vi "Sort DPID IDs by Speed.vi"(11 "DPIDs":T2[](array[typedef])) -> (3 "Filtered DPIDs IDs":T1)   [LabVIEW 2013]
uses:
  DPID Parameters.ctl
  DPID Periodic Rate.ctl
  Filtered DPID IDs.ctl
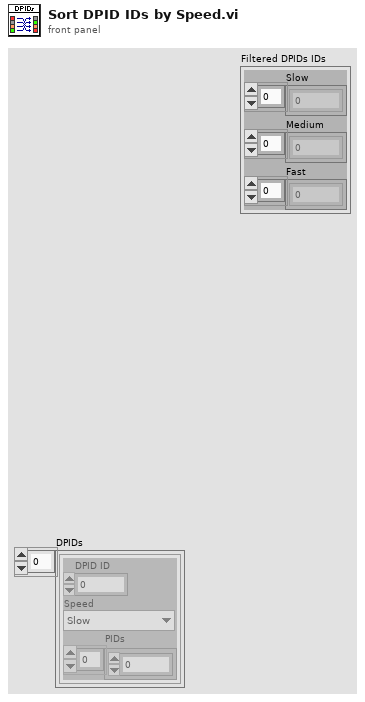
[diagram p1: front panel]
types:
  T1 = typedef "Filtered DPID IDs.ctl" = cluster{"Slow":u8[], "Medium":u8[], "Fast":u8[]}
  T2 = typedef "DPID Parameters.ctl" = cluster{"DPID ID":u8, "Speed":T3, "PIDs":u16[]}
  T3 = typedef "DPID Periodic Rate.ctl" = enum16{"Slow", "Medium", "Fast"}
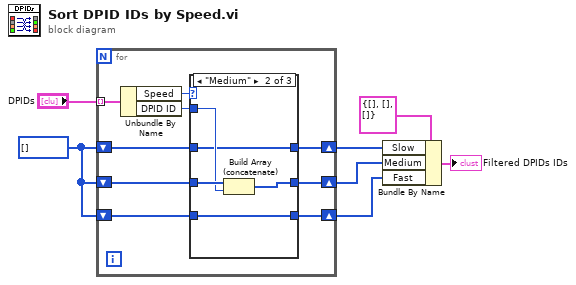
[diagram p0: block diagram]
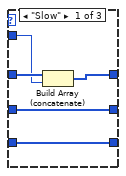
[diagram p2: hidden frame]
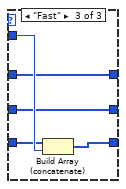
[diagram p3: hidden frame]
diagram:
  w6 = u8[] []
  n1 = for {
    tunnel: "DPIDs" -> [w16] mode=indexing
    shift-right: [w8] -> w5
    shift-left: w6 -> [w14]
    shift-right: [w12] -> w4
    shift-left: w6 -> [w11]
    shift-right: [w10] -> w3
    shift-left: w6 -> [w9]
    n2 = Unbundle By Name(w16) -> ("Speed"=w15:T3, "DPID ID"=w13:u8)
    n3 = case shown="\"Medium\"" w15 {
      tunnel: w14 -> [w21 w23 w30]
      tunnel: w13 -> [w20 w25 w31]
      tunnel: [w19 w24 w29] -> w12
      tunnel: w11 -> [w19 w26 w29]
      tunnel: [w18 w22 w27] -> w10
      tunnel: w9 -> [w18 w22 w28]
      tunnel: [w17 w23 w30] -> w8
      frame "Slow" {
        n4 = Build Array (concatenate)(w21, w20) -> (w17:u8[])
      }
      frame "Medium" {
        n5 = Build Array (concatenate)(w26, w25) -> (w24:u8[])
      }
      frame "Fast" {
        n6 = Build Array (concatenate)(w28, w31) -> (w27:u8[])
      }
    }
  }
  n7 = Bundle By Name(cluster=T1 {"Slow"=[], "Medium"=[], "Fast"=[]}, "Slow"=w5, "Medium"=w4, "Fast"=w3) -> (→"Filtered DPIDs IDs":T1)
